vi "main.vi"(8 "错误常量":errorcluster) -> (0 "error out":errorcluster)   [LabVIEW 2015, in "Browse.lvlib"]
uses:
  Browse.lvlib
  Support/Browse UI Data.ctl
  <vilib>/addons/database/Connection.llb/Conn ObjectReference.ctl
  Support/Main State.ctl
  <vilib>/addons/database/NI_Database_API.lvlib
  Sub VIs/Database Processing/Database Processing.lvlib
  Sub VIs/Utility VIs/Utility VIs.lvlib
panel:
  out "排列表格":string[][](table)
  in  "患者名字":string
  in  "患者编号":i64
  out "患者眼球测量结果":string[][](table)
  in  "停止按钮":bool
  out "状态栏":string
  # "患者眼球参数浏览"
  # "患者眼球测量结果"
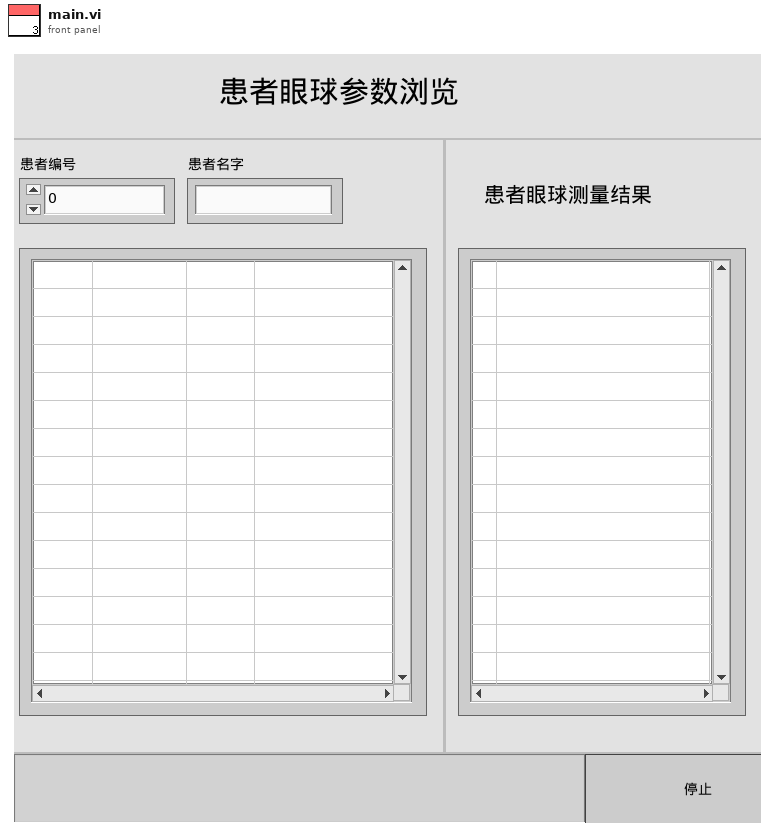
[diagram p1: front panel]
types:
  T1 = typedef "Browse.lvlib/Main State.ctl" = enum16{"Initialize", "Connect Database", "Update Personal Information", "Update Measure Bio Type", "Update Biometry Average", "Wait For Event", "Exit"}
  T2 = typedef "NI_Database_API.lvlib/Conn ObjectReference.ctl" = refnum<k1>
  T3 = typedef "Browse.lvlib/Browse UI Data.ctl" = cluster{"患者编号引用句柄":refnum<vi>, "患者名字引用句柄":refnum<vi>, "排列表格引用句柄":refnum<vi>, "患者眼球测量结果引用句柄 ":refnum<vi>, "状态栏引用句柄":refnum<vi>, "Bool引用句柄":refnum<vi>}
  T4 = typedef "LVPoint32TypeDef.ctl" = cluster{"Horizontal":i32, "Vertical":i32}
  T5 = typedef "LVRowAndColumnTypeDef.ctl" = cluster{"Row":i32, "Column":i32}
  T6 = typedef "Database Processing.lvlib/personal_information.ctl" = cluster{"Patient_ID":i64, "name":string, "sex":string, "birthday":string}
  T7 = typedef "Database Processing.lvlib/Measure_Bio_Type.ctl" = cluster{"Measure_No":i64, "Measure_Time":string, "Patient_ID":i64}
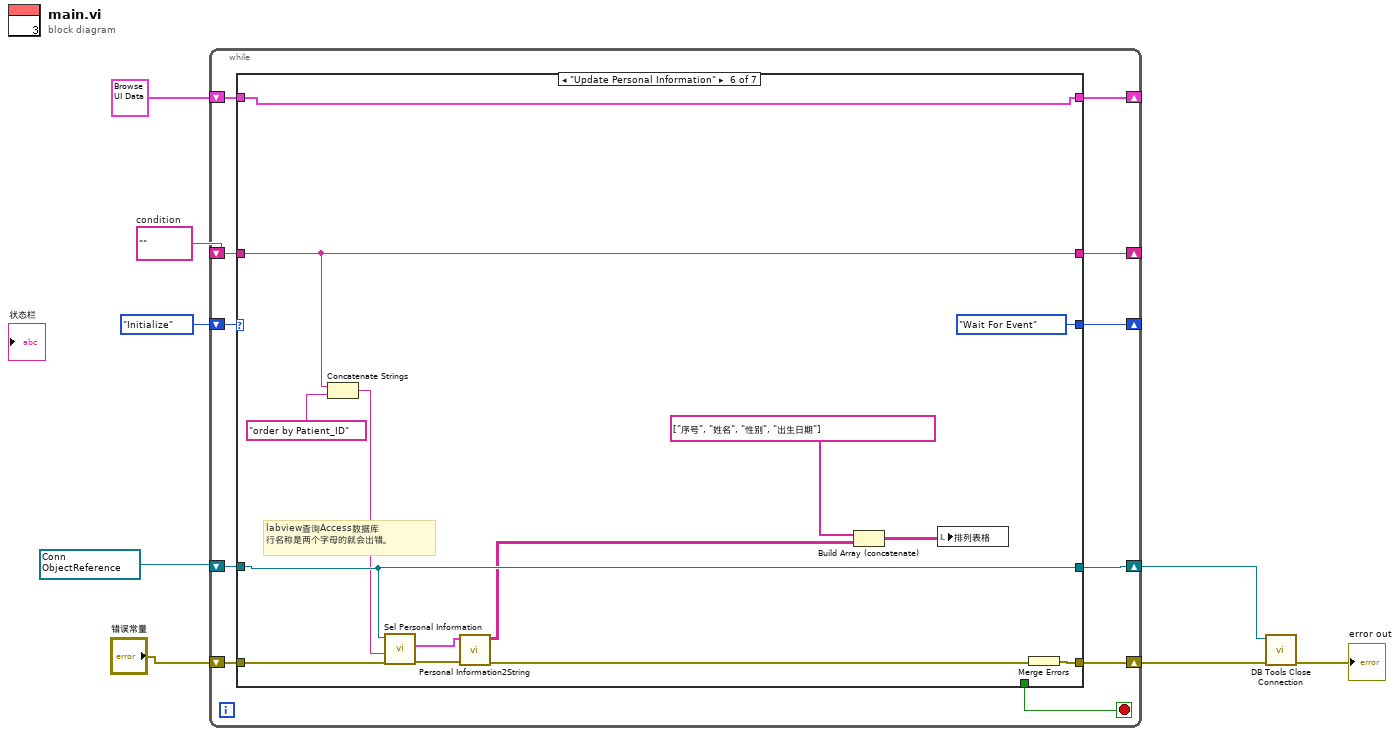
[diagram p0: block diagram]
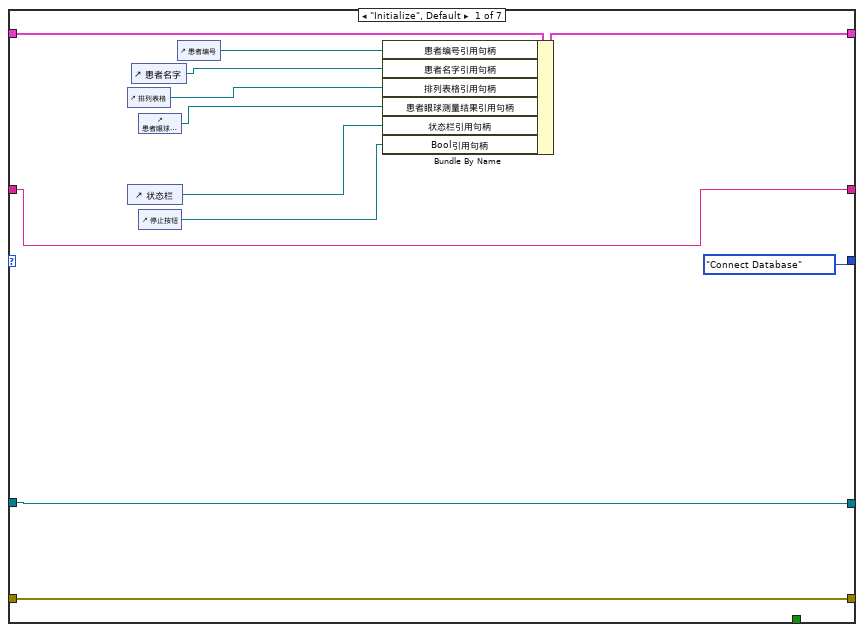
[diagram p2: hidden frame]
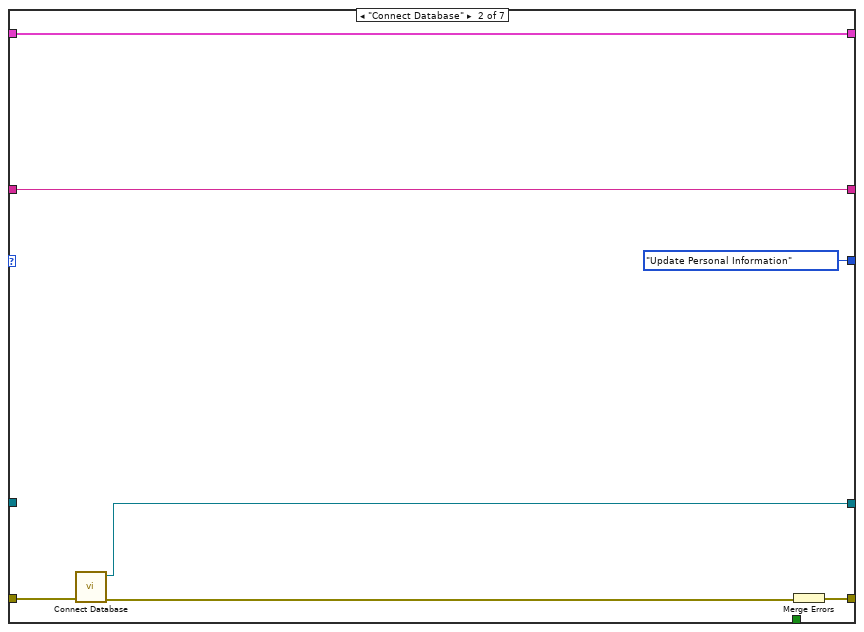
[diagram p3: hidden frame]
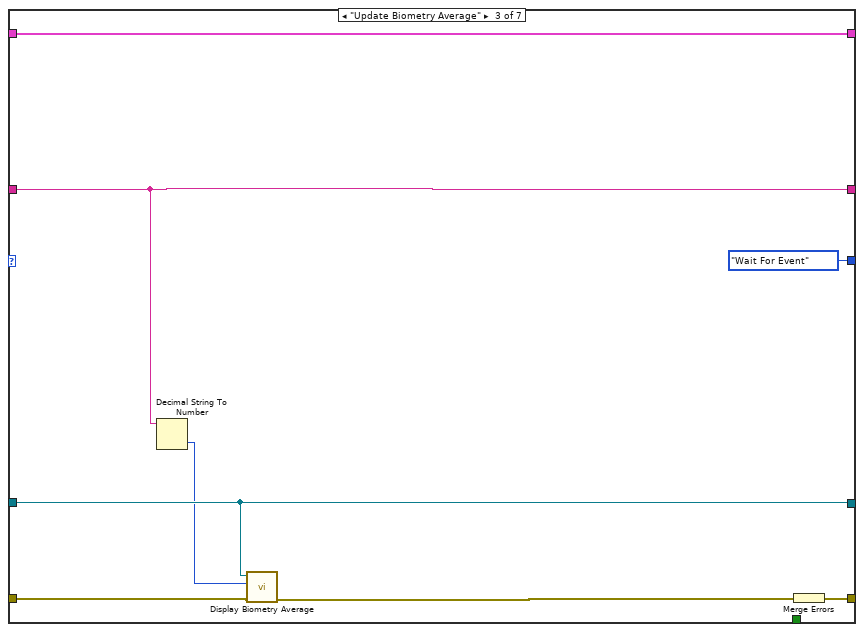
[diagram p4: hidden frame]
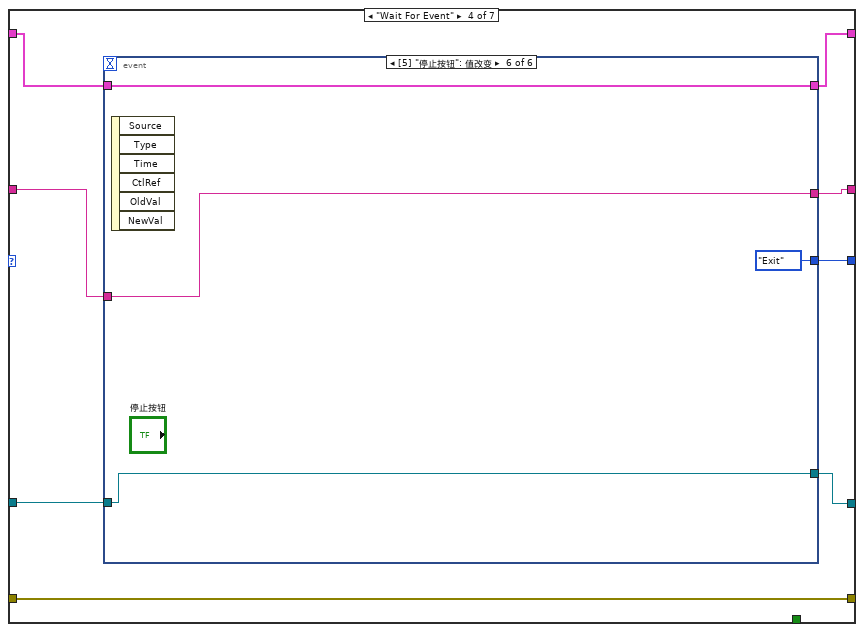
[diagram p5: hidden frame]
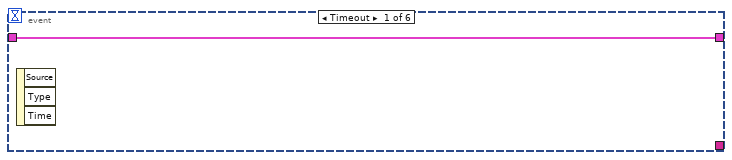
[diagram p6: hidden frame]
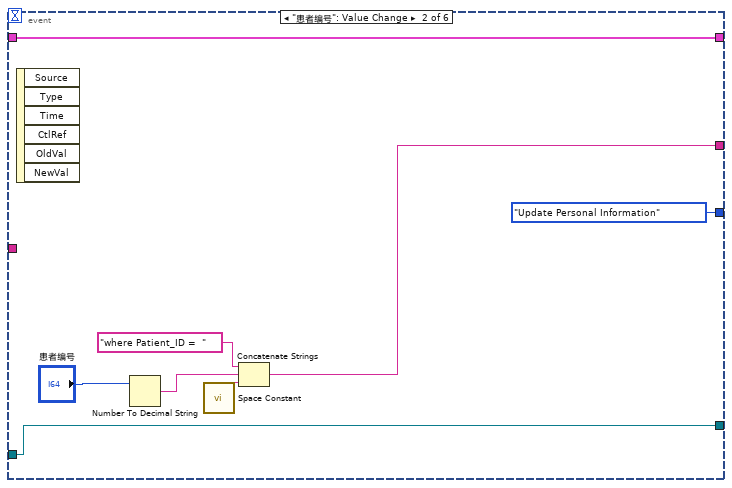
[diagram p7: hidden frame]
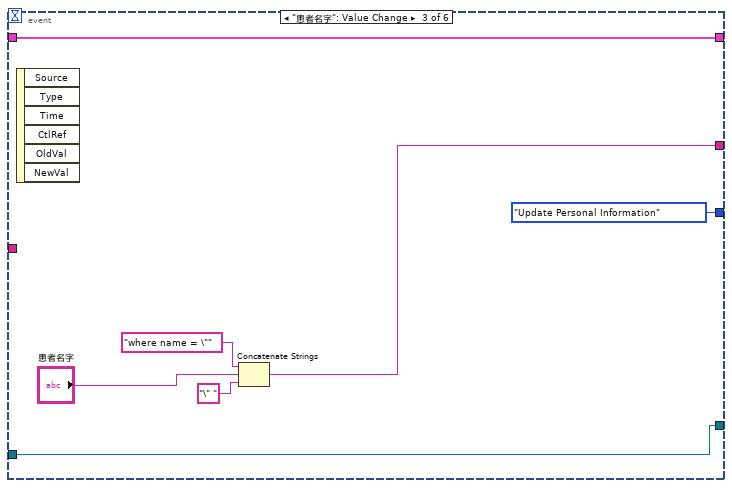
[diagram p8: hidden frame]
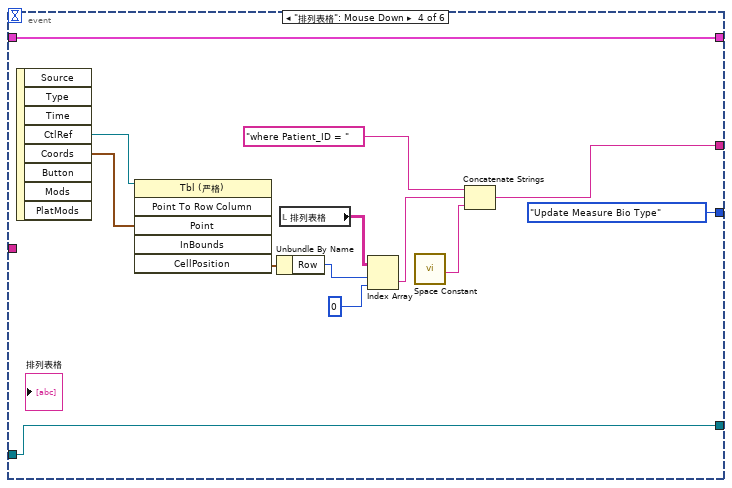
[diagram p9: hidden frame]
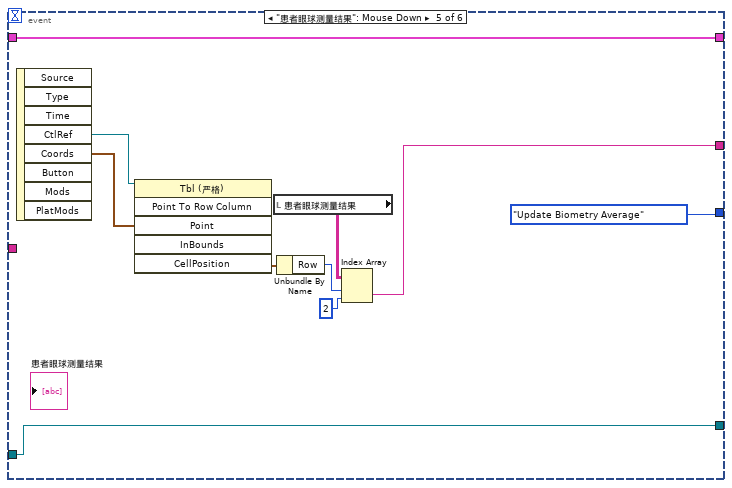
[diagram p10: hidden frame]
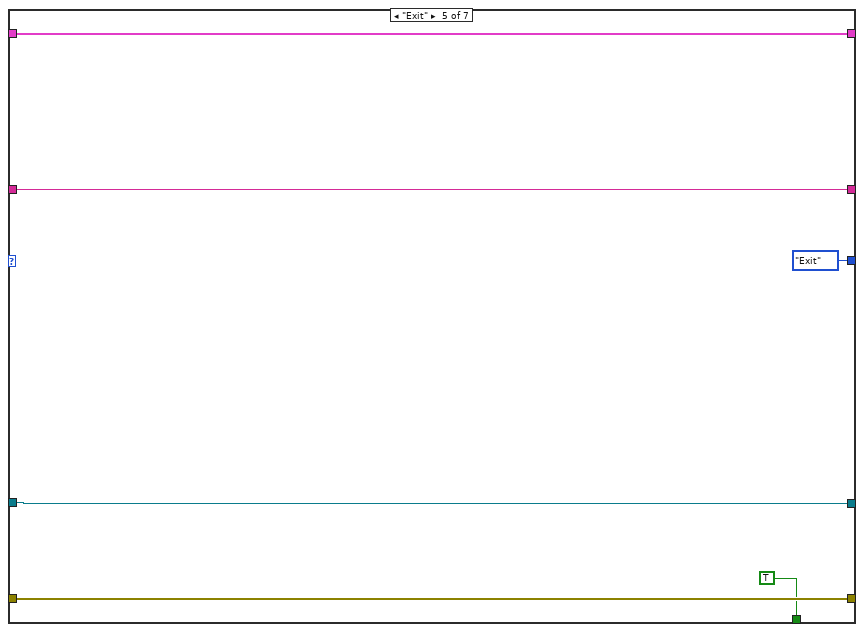
[diagram p11: hidden frame]
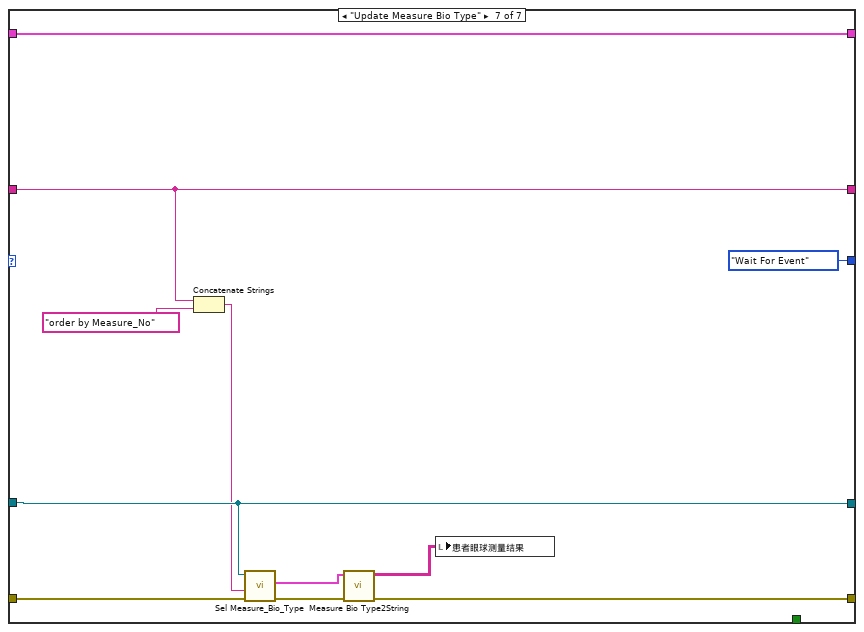
[diagram p12: hidden frame]
diagram:
  w4 = ""  # condition
  w5 = T2 refnum items=["Connection"] ("connection reference")
  n1 = while {
    shift-right: [w18] -> _
    shift-left: T3 {"患者编号引用句柄"=refnum, "患者名字引用句柄"=refnum, "排列表格引用句柄"=refnum, "患者眼球测量结果引用句柄 "=refnum, "状态栏引用句柄"=refnum, "Bool引用句柄"=refnum} ("UI数据") -> [w19]
    shift-right: [w10] -> _
    shift-left: Main_State."Initialize" ("State") -> [w9]
    shift-right: [w15] -> w7
    shift-left: "错误常量" -> [w17]
    shift-right: [w13] -> _
    shift-left: w4 -> [w16]
    shift-right: [w12] -> w3
    shift-left: w5 -> [w11]
    stop <- w14 stop-if-true
    n2 = case shown="\"Update Personal Information\"" w9 {
      tunnel: w19 -> [w31 w33 w45 w51 w103 w114 w128]
      tunnel: [w27 w33 w45 w50 w103 w114 w128] -> w18
      tunnel: [Main_State."Connect Database" ("State") Main_State."Update Personal Information" ("State") Main_State."Wait For Event" ("State") w47 Main_State."Exit" ("State") Main_State."Wait For Event" ("State") Main_State."Wait For Event" ("State")] -> w10
      tunnel: w17 -> [w26 w37 w44 w52 w101 w113 w127]
      tunnel: w16 -> [w25 w34 w41 w54 w102 w110 w125]
      tunnel: [w26 w38 w46 w52 w101 w115 w121] -> w15
      tunnel: [w25 w34 w41 w53 w102 w110 w125] -> w13
      tunnel: [_ _ _ _ TRUE _ _] -> w14
      tunnel: w11 -> [w21 _ w42 w49 w100 w112 w126]
      tunnel: [w21 w35 w42 w48 w100 w112 w126] -> w12
      frame "Initialize", Default {
        n3 = control-ref of="排列表格"() -> (w28:refnum<vi>)
        n4 = control-ref of="状态栏"() -> (w23:refnum<vi>)
        n5 = control-ref of="患者名字"() -> (w29:refnum<vi>)
        n6 = control-ref of="患者眼球测量结果"() -> (w24:refnum<vi>)
        n7 = control-ref of="停止按钮"() -> (w22:refnum<vi>)
        n8 = control-ref of="患者编号"() -> (w30:refnum<vi>)
        n9 = Bundle By Name(cluster=w31, "患者编号引用句柄"=w30, "患者名字引用句柄"=w29, "排列表格引用句柄"=w28, "患者眼球测量结果引用句柄"=w24, "状态栏引用句柄"=w23, "Bool引用句柄"=w22) -> (w27:T3)
      }
      frame "Connect Database" {
        n10 = call "Connect Database.vi"("error in (no error)"=w37) -> ("error out"=w36:errorcluster, "connection reference"=w35:T2)  [unwired: 9 in]
        n11 = Merge Errors(w36) -> (w38:errorcluster)
      }
      frame "Update Biometry Average" {
        n12 = Decimal String To Number(string=w41) -> (number=w40:i32)  [unwired: 2 in, 1 out]
        n13 = call "Display Biometry Average.vi"("错误常量 2"=w44, "Measure_No"=w40, "connection reference"=w42) -> ("错误常量"=w43:errorcluster)  [unwired: 8 in]
        n14 = Merge Errors(w43) -> (w46:errorcluster)
      }
      frame "Wait For Event" {
        n15 = event shown="[5] \"停止按钮\": 值改变" {
          selector: _ -> [_ _ _ _ _ _]
          dyn-events: _ -> [_ _ _ _ _ _]
          timeout: _ -> [_ _ _ _ _ _]
          tunnel: w54 -> [_ _ _ _ _ w97]
          tunnel: [_ w58 w65 w73 w85 w97] -> w53
          tunnel: [_ Main_State."Update Personal Information" ("State") Main_State."Update Personal Information" ("State") Main_State."Update Measure Bio Type" ("State") Main_State."Update Biometry Average" ("State") Main_State."Exit" ("State")] -> w47
          tunnel: w51 -> [w55 w60 w67 w76 w88 w96]
          tunnel: [w55 w60 w67 w76 w88 w96] -> w50
          tunnel: w49 -> [_ w59 w66 w74 w86 w95]
          tunnel: [_ w59 w66 w74 w86 w95] -> w48
          event Timeout {
            n16 = event-data() -> ()  [unwired: 1 in, 3 out]
          }
          event "患者编号": Value Change {
            n17 = event-data() -> ()  [unwired: 1 in, 6 out]
            n18 = Number To Decimal String(number="患者编号") -> (decimal integer string=w61:string)  [unwired: 1 in]
            n19 = call <vilib>:"Space Constant.vi"() -> ("String"=w57:string)
            n20 = Concatenate Strings("where Patient_ID =  " ("字符串"), w61, w57) -> (w58:string)
          }
          event "患者名字": Value Change {
            n21 = event-data() -> ()  [unwired: 1 in, 6 out]
            n22 = Concatenate Strings("where name = \"" ("字符串"), "患者名字", "\" " ("字符串")) -> (w65:string)
          }
          event "排列表格": Mouse Down {
            n23 = event-data() -> ("CtlRef"=w75:refnum<vi>, "Coords"=w83:T4)  [unwired: 1 in, 6 out]
            n24 = invoke on="调用节点" class="Tbl (严格)" method="Point To Row Column"(reference=w75, "Point"=w83) -> ("CellPosition"=w82:T5)  [unwired: 4 in, 5 out]
            n25 = Unbundle By Name(w82) -> ("Row"=w81:i32)
            n26 = local read "排列表格"() -> (w80:string[][])
            n27 = Index Array(array=w80, index (row)=w81, index (col)=0 ("禁用的索引 (列)")) -> (element=w77:string)
            n28 = call <vilib>:"Space Constant.vi"() -> ("String"=w72:string)
            n29 = Concatenate Strings("where Patient_ID = " ("字符串"), w77, w72) -> (w73:string)
          }
          event "患者眼球测量结果": Mouse Down {
            n30 = event-data() -> ("CtlRef"=w87:refnum<vi>, "Coords"=w93:T4)  [unwired: 1 in, 6 out]
            n31 = invoke on="调用节点" class="Tbl (严格)" method="Point To Row Column"(reference=w87, "Point"=w93) -> ("CellPosition"=w92:T5)  [unwired: 4 in, 5 out]
            n32 = local read "患者眼球测量结果"() -> (w90:string[][])
            n33 = Unbundle By Name(w92) -> ("Row"=w91:i32)
            n34 = Index Array(array=w90, index (row)=w91, index (col)=2 ("禁用的索引 (列)")) -> (element=w85:string)
          }
          event "停止按钮": Value Change {
            n35 = event-data() -> ()  [unwired: 1 in, 6 out]
          }
        }
      }
      frame "Exit" {
      }
      frame "Update Personal Information" {
        # "labview查询Access数据库\n行名称是两个字母的就会出错。"
        n36 = Concatenate Strings(w110, "order by Patient_ID" ("字符串")) -> (w111:string)
        n37 = call "Sel Personal Information.vi"("error in (no error)"=w113, "condition"=w111, "connection reference"=w112) -> ("error out"=w108:errorcluster, "personal information"=w107:T6[])  [unwired: 7 in]
        n38 = call "Personal Information2String.vi"("error in (no error)"=w108, "personal information"=w107) -> ("error out"=w105:errorcluster, "personal information"=w106:string[][])  [unwired: 8 in]
        n39 = Build Array (concatenate)(string[] ["序号", "姓名", "性别", "出生日期"], w106) -> (w116:string[][])
        n40 = local write "排列表格"(w116) -> ()
        n41 = Merge Errors(w105) -> (w115:errorcluster)
      }
      frame "Update Measure Bio Type" {
        n42 = Concatenate Strings(w125, "order by Measure_No" ("字符串")) -> (w124:string)
        n43 = call "Sel Measure_Bio_Type.vi"("error in (no error)"=w127, "condition"=w124, "connection reference"=w126) -> ("error out"=w122:errorcluster, "Measure_Bio_Typea"=w120:T7[])  [unwired: 7 in]
        n44 = call "Measure Bio Type2String.vi"("error in (no error)"=w122, "Measure_Bio_Type Input"=w120) -> ("error out"=w121:errorcluster, "Measure Bio Type"=w119:string[][])  [unwired: 8 in]
        n45 = local write "患者眼球测量结果"(w119) -> ()
      }
    }
  }
  n46 = call <vilib>:"DB Tools Close Connection.vi"("error in (no error)"=w7, "connection reference"=w3) -> ("error out"=→"error out":errorcluster)  [unwired: 5 in]
